vi "inclineCount.vi"(8 "error in (no error)":errorcluster, 10 "negative incline":dbl, 11 "max incline":dbl) -> (0 "error out":errorcluster, 1 "press start":dbl, 2 "max incline":dbl, 3 "count incline":i32)   [LabVIEW 2018]
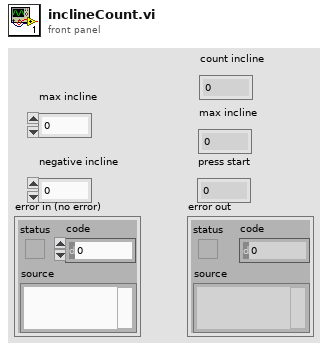
[diagram p1: front panel]
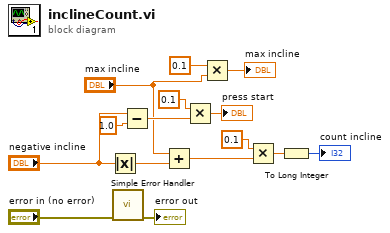
[diagram p0: block diagram]
diagram:
  n1 = Absolute Value(x="negative incline") -> (abs(x)=w10:dbl)
  n2 = call <vilib>:"Simple Error Handler.vi"("error in (no error)"="error in (no error)") -> ("error out"=→"error out":errorcluster)  [unwired: 4 in, 4 out]
  n3 = Subtract(x="negative incline", y=1.0) -> (x-y=w13:dbl)
  n4 = Add(x="max incline", y=w10) -> (x+y=w6:dbl)
  n5 = Multiply(x=0.1, y=w13) -> (x*y=→"press start":dbl)
  n6 = Multiply(x=0.1, y="max incline") -> (x*y=→"max incline":dbl)
  n7 = Multiply(x=0.1, y=w6) -> (x*y=w8:dbl)
  n8 = To Long Integer(number=w8) -> (32bit integer=→"count incline":i32)
